vi "Update image if new.vi"(0 "Raw images":T1[](array[typedef]), 1 "Image Dst":T1, 2 "DownloadedImg":T1, 3 "USB cameras":i32, 4 "Buffer2":T1) -> (5 "Image Dst Out":T1, 6 "Image ok":bool)   [LabVIEW 2013]
uses:
  <vilib>/vision/Image Controls.llb/IMAQ Image.ctl
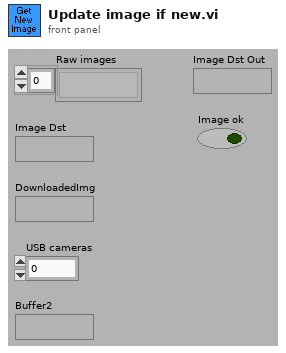
[diagram p1: front panel]
types:
  T1 = typedef "IMAQ Image.ctl" = refnum<image>
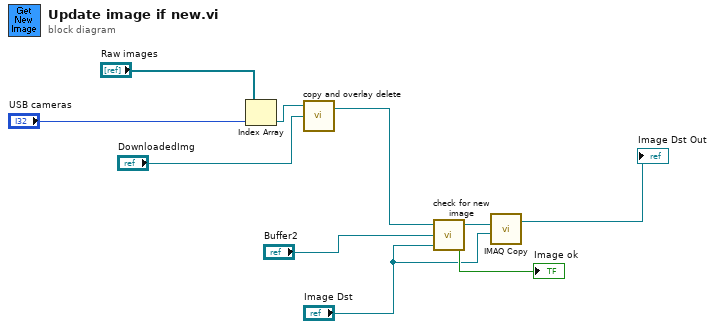
[diagram p0: block diagram]
diagram:
  n1 = Index Array(array="Raw images", index="USB cameras") -> (element=w7:T1)
  n2 = call "copy and overlay delete.vi"("Image Dst"="DownloadedImg", "Image in"=w7) -> ("Image Out"=w8:T1)  [unwired: 1 in, 1 out]
  n3 = call "check for new image.vi"("Acq Img"="Image Dst", "Buffer"="Buffer2", "Downloaded image"=w8) -> ("Image ok"=→"Image ok":bool, "Image Out"=w9:T1)  [unwired: 1 out]
  n4 = call "IMAQ Copy"("Image Dst"="Image Dst", "Image Src"=w9) -> ("Image Dst Out"=→"Image Dst Out":T1)  [unwired: 4 in, 1 out]
